vi "FindIndexofStringInstringArray.vi"(8 "error in (no error)":errorcluster, 10 "Searched String":string, 11 "String Array input":string[](array[string])) -> (0 "error out":errorcluster, 1 "BeforeEqualSignString":string, 2 "AfterEqualSignString":string, 3 "String Array outpu":string[](array[string]))   [LabVIEW 2017]
doc: "Use this template to build a VI to use as a subVI."
uses:
  <vilib>/regexp/Match Regular Expression.xnode
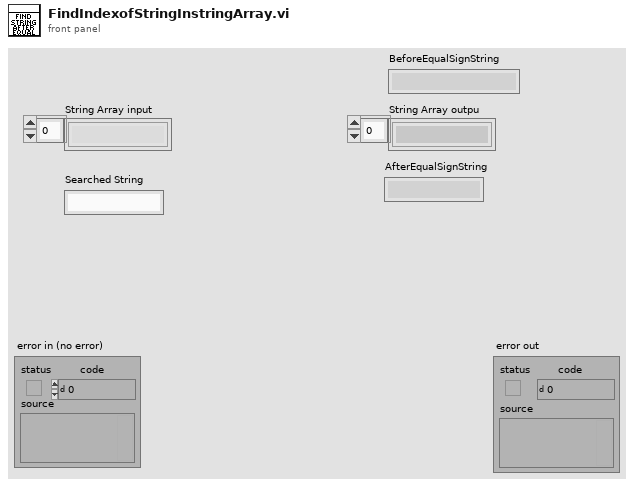
[diagram p1: front panel]
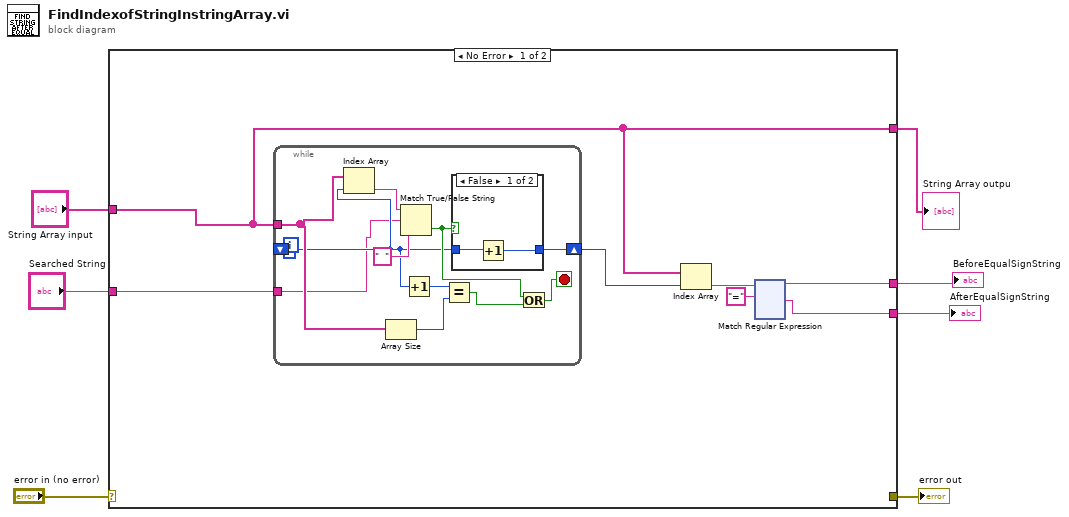
[diagram p0: block diagram]
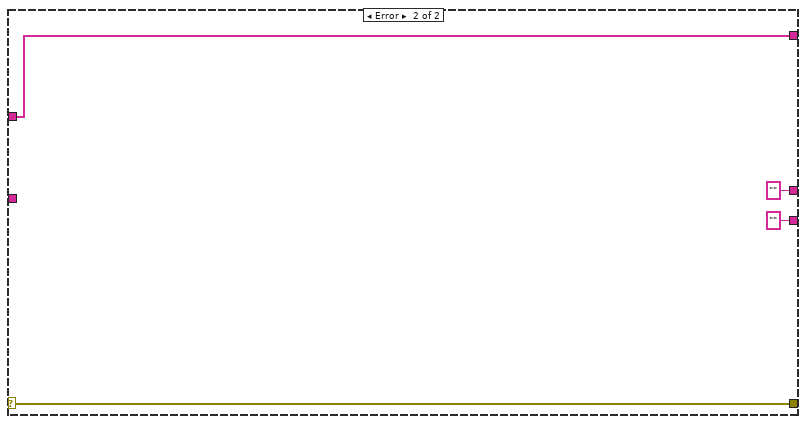
[diagram p3: hidden frame]
diagram:
  n1 = case shown="No Error" "error in (no error)" {
    selector: "error in (no error)" -> [_ w147]
    tunnel: [_ w147] -> w6
    tunnel: "String Array input" -> [w10 w146]
    tunnel: "Searched String" -> [w14 _]
    tunnel: [w10 w146] -> w3
    tunnel: [w9 "" ("after match")] -> w2
    tunnel: [w8 "" ("before match")] -> w1
    frame No Error {
      n2 = while {
        shift-right: [w140] -> w11
        shift-left: 0 -> [w134]
        tunnel: w10 -> [w136]
        tunnel: w14 -> [w130]
        stop <- w131 stop-if-true
        n3 = Index Array(array=w136, index=w134) -> (element=w139:string)
        n4 = Array Size(array=w136) -> (size(s)=w133:i32)
        n5 = Match True/False String(2:"  " ("false string"), 3:w130, 4:w139) -> (0:w137:bool)  [unwired: 1 out]
        n6 = Increment(x=w134) -> (x+1=w135:i32)
        n7 = Equal?(x=w135, y=w133) -> (x = y?=w132:bool)
        n8 = case shown="False" w137 {
          tunnel: w134 -> [w142 w143]
          tunnel: [w141 w143] -> w140
          frame False {
            n9 = Increment(x=w142) -> (x+1=w141:i32)
          }
          frame True {
          }
        }
        n10 = Or(x=w137, y=w132) -> (x .or. y?=w131:bool)
      }
      n11 = Index Array(array=w10, index=w11) -> (element=w13:string)
      n12 = xnode "Match Regular Expression"("input string"=w13, "regular expression"="=") -> ("before match"=w8:string, "after match"=w9:string)  [unwired: 4 in, 3 out]
    }
    frame Error {
    }
  }
  "error out" <- w6
  "String Array outpu" <- w3
  "AfterEqualSignString" <- w2
  "BeforeEqualSignString" <- w1
